vi "ConfigureSweep.vi"(4 "FullScaleVoltage":dbl=800.0, 6 "DetectionMode":enum16{"Peak", "Quasi Peak", "Average"}(ring), 8 "error in (no error)":errorcluster, 9 "DetectionTime":dbl=0.01 format="%#_6p", 10 "Sweep":cluster{"Center Freq":dbl, "Bandwidth":dbl}[](array[cluster]), 11 "9770 API in":refnum<class "9770 API.lvclass">) -> (0 "error out":errorcluster, 3 "9770 API out":refnum<class "9770 API.lvclass">)   [LabVIEW 2017, in "9770 API.lvclass"]
uses:
  <vilib>/addons/InsightCM/Devices/Shared/Emsa/Emsa9770API/9770 API.lvclass
  <vilib>/addons/InsightCM/Devices/Shared/Emsa/Emsa9770API/9770 API.lvclass/9770 API.ctl
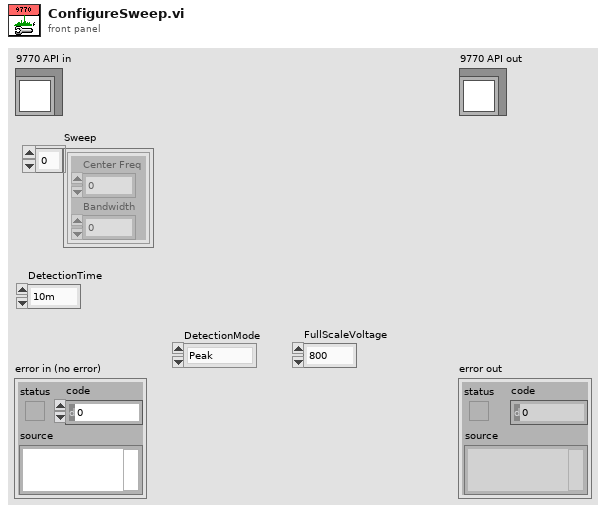
[diagram p1: front panel]
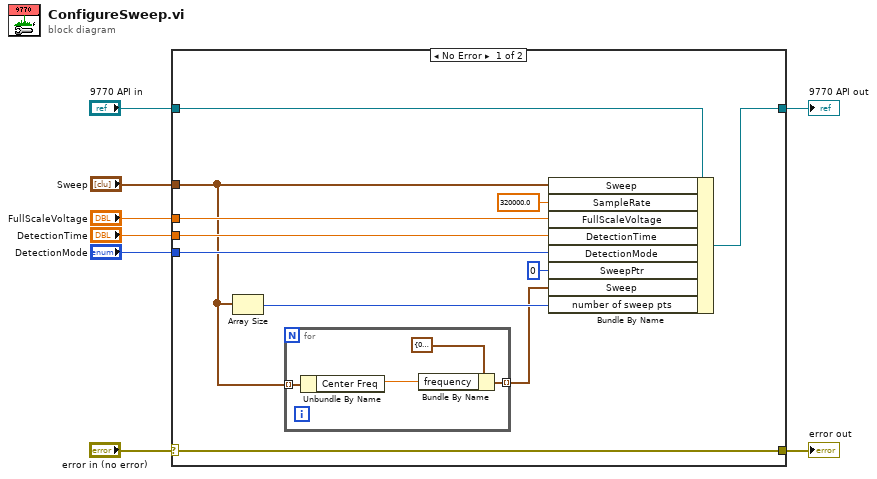
[diagram p0: block diagram]
diagram:
  n1 = case shown="No Error" "error in (no error)" {
    selector: "error in (no error)" -> [w19 w25]
    tunnel: [w19 w25] -> w7
    tunnel: [w17 w24] -> w5
    tunnel: "9770 API in" -> [w18 w24]
    tunnel: "Sweep" -> [w10 _]
    tunnel: "FullScaleVoltage" -> [w16 _]
    tunnel: "DetectionTime" -> [w15 _]
    tunnel: "DetectionMode" -> [w14 _]
    frame No Error {
      n2 = Array Size(array=w10) -> (size(s)=w11:i32)
      n3 = for {
        tunnel: w10 -> [w23] mode=indexing
        tunnel: [w20] -> w9 mode=indexing
        n4 = Unbundle By Name(w23) -> ("Center Freq"=w21:dbl)
        n5 = Bundle By Name(cluster=cluster{"frequency":dbl, "amplitude":dbl} {"frequency"=0.0, "amplitude"=0.0} ("sweep"), "frequency"=w21) -> (w20:cluster{"frequency":dbl, "amplitude":dbl})
      }
      n6 = Bundle By Name(cluster=w18, "Sweep"=w10, "SampleRate"=320000.0 ("SweepCfg.SampleRate"), "FullScaleVoltage"=w16, "DetectionTime"=w15, "DetectionMode"=w14, "SweepPtr"=0 ("state.SweepPtr"), "Sweep"=w9, "number of sweep pts"=w11) -> (w17:refnum<class "9770 API.lvclass">)
    }
    frame Error {
    }
  }
  "error out" <- w7
  "9770 API out" <- w5
